vi "试剂余量显示UI.vi"() -> ()   [LabVIEW 2016, in "斯坦道CODMn新电路板.lvlib"]
uses:
  <vilib>/Utility/miscctls.llb/LVPointTypeDef.ctl
panel:
  in  "余量 14":string
  in  "余量 13":string
  in  "余量 12":string
  in  "余量 11":string
  in  "余量 10":string
  in  "余量 9":string
  in  "余量 8":string
  in  "余量 7":string
  in  "余量 6":string
  in  "余量 5":string
  in  "余量 4":string
  in  "余量 3":string
  in  "余量 2":string
  in  "余量":string
  in  "关闭":bool
  in  "全部重置":bool
  in  "试剂容量设置":bool
  in  "试剂名称设置":bool
  in  "重置 14":bool
  out "试剂 14":dbl(slide) caption="V9-2.试剂14" scale=0.0..100.0 scale format="%#_f %%"
  in  "重置 13":bool
  out "试剂 13":dbl(slide) caption="V9-1.试剂13" scale=0.0..100.0 scale format="%#_f %%"
  in  "重置 12":bool
  out "试剂 12":dbl(slide) caption="V12.试剂12" scale=0.0..100.0 scale format="%#_f %%"
  in  "重置 11":bool
  out "试剂 11":dbl(slide) caption="V11.试剂11" scale=0.0..100.0 scale format="%#_f %%"
  in  "重置 10":bool
  out "试剂 10":dbl(slide) caption="V10.试剂10" scale=0.0..100.0 scale format="%#_f %%"
  in  "重置 9":bool
  out "试剂 9":dbl(slide) caption="V9.试剂9" scale=0.0..100.0 scale format="%#_f %%"
  in  "重置 8":bool
  out "试剂 8":dbl(slide) caption="V8.试剂8" scale=0.0..100.0 scale format="%#_f %%"
  in  "重置 7":bool
  out "试剂 7":dbl(slide) caption="V7.试剂7" scale=0.0..100.0 scale format="%#_f %%"
  in  "重置 6":bool
  out "试剂 6":dbl(slide) caption="V6.试剂6" scale=0.0..100.0 scale format="%#_f %%"
  in  "重置 5":bool
  out "试剂 5":dbl(slide) caption="V5.试剂5" scale=0.0..100.0 scale format="%#_f %%"
  in  "重置 4":bool
  out "试剂 4":dbl(slide) caption="V4.试剂4" scale=0.0..100.0 scale format="%#_f %%"
  in  "重置 3":bool
  out "试剂 3":dbl(slide) caption="V3.试剂3" scale=0.0..100.0 scale format="%#_f %%"
  in  "重置 2":bool
  out "试剂 2":dbl(slide) caption="V2.试剂2" scale=0.0..100.0 scale format="%#_f %%"
  in  "重置":bool
  out "试剂":dbl(slide) caption="V1.试剂1" scale=0.0..100.0 scale format="%#_f %%"
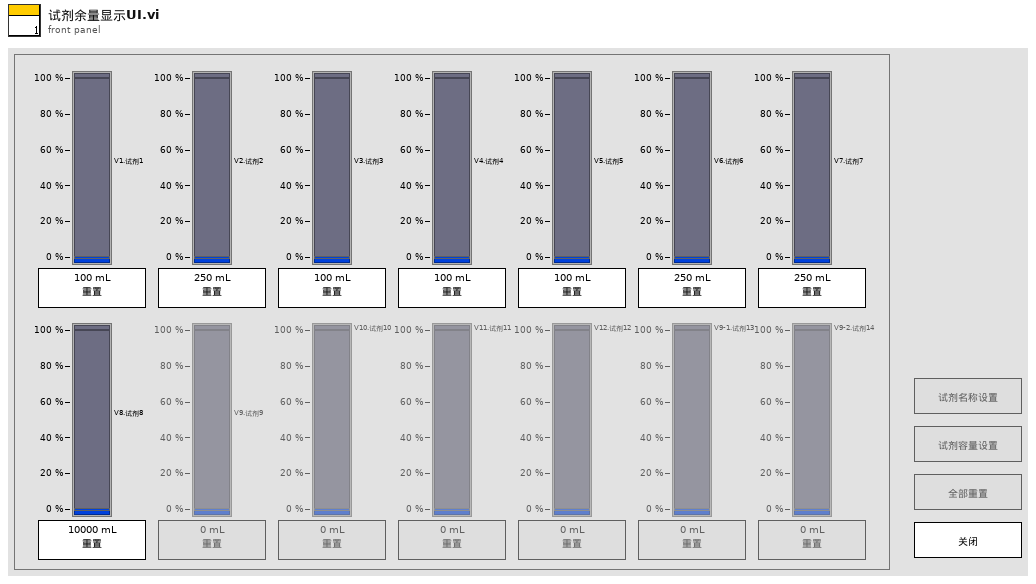
[diagram p1: front panel]
types:
  T1 = typedef "LVPointTypeDef.ctl" = cluster{"Horizontal":i16, "Vertical":i16}
  T2 = enum8{"Enabled", "Disabled", "Disabled and Grayed Out"}
  T3 = cluster{"时间标识":timestamp, "设备":string, "日志信息":string, "流程参数":string}
  T4 = cluster{"V1":sgl, "V2":sgl, "V3":sgl, "V4":sgl, "V5":sgl, "V6":sgl, "V7":sgl, "V8":sgl, "V9":sgl, "V10":sgl, "V11":sgl, "V12":sgl, "V9-1":sgl, "V9-2":sgl}
  T5 = cluster{"V":string, "V 2":string, "V 3":string, "V 4":string, "V 5":string, "V 6":string, "V 7":string, "V 8":string, "V 9":string, "V 10":string, "V 11":string, "V 12":string, "V9-1":string, "V9-2":string}
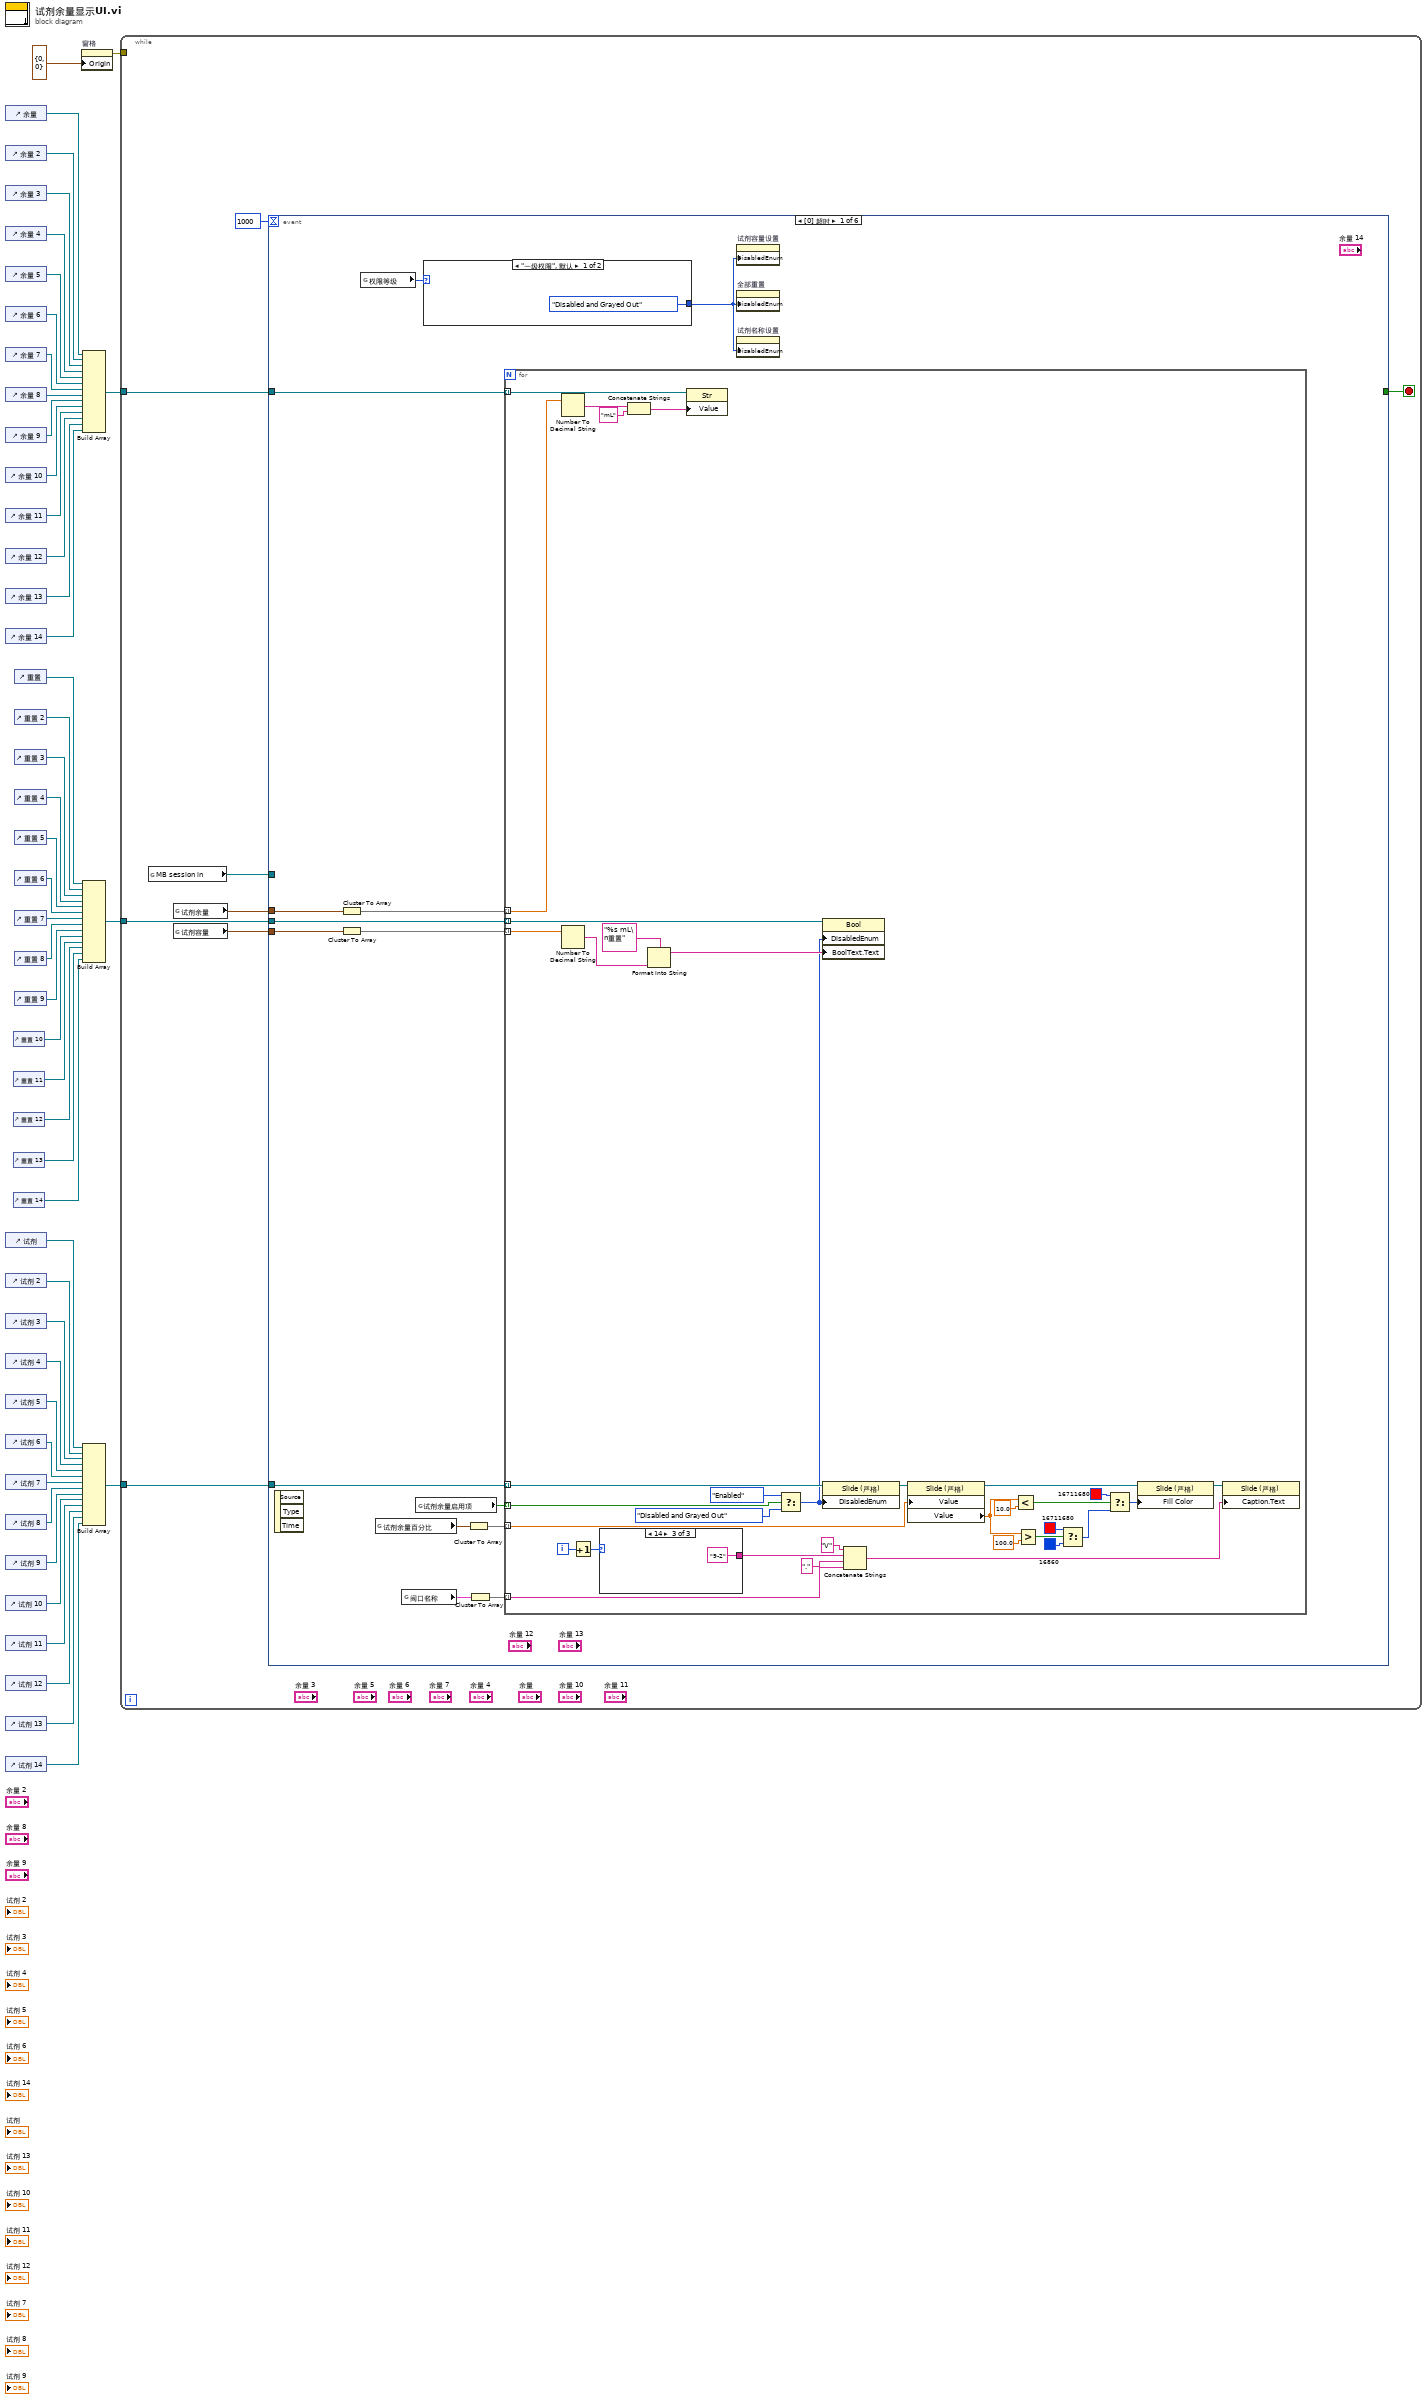
[diagram p0: block diagram]
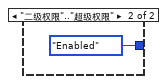
[diagram p2: hidden frame]
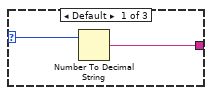
[diagram p3: hidden frame]
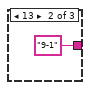
[diagram p4: hidden frame]
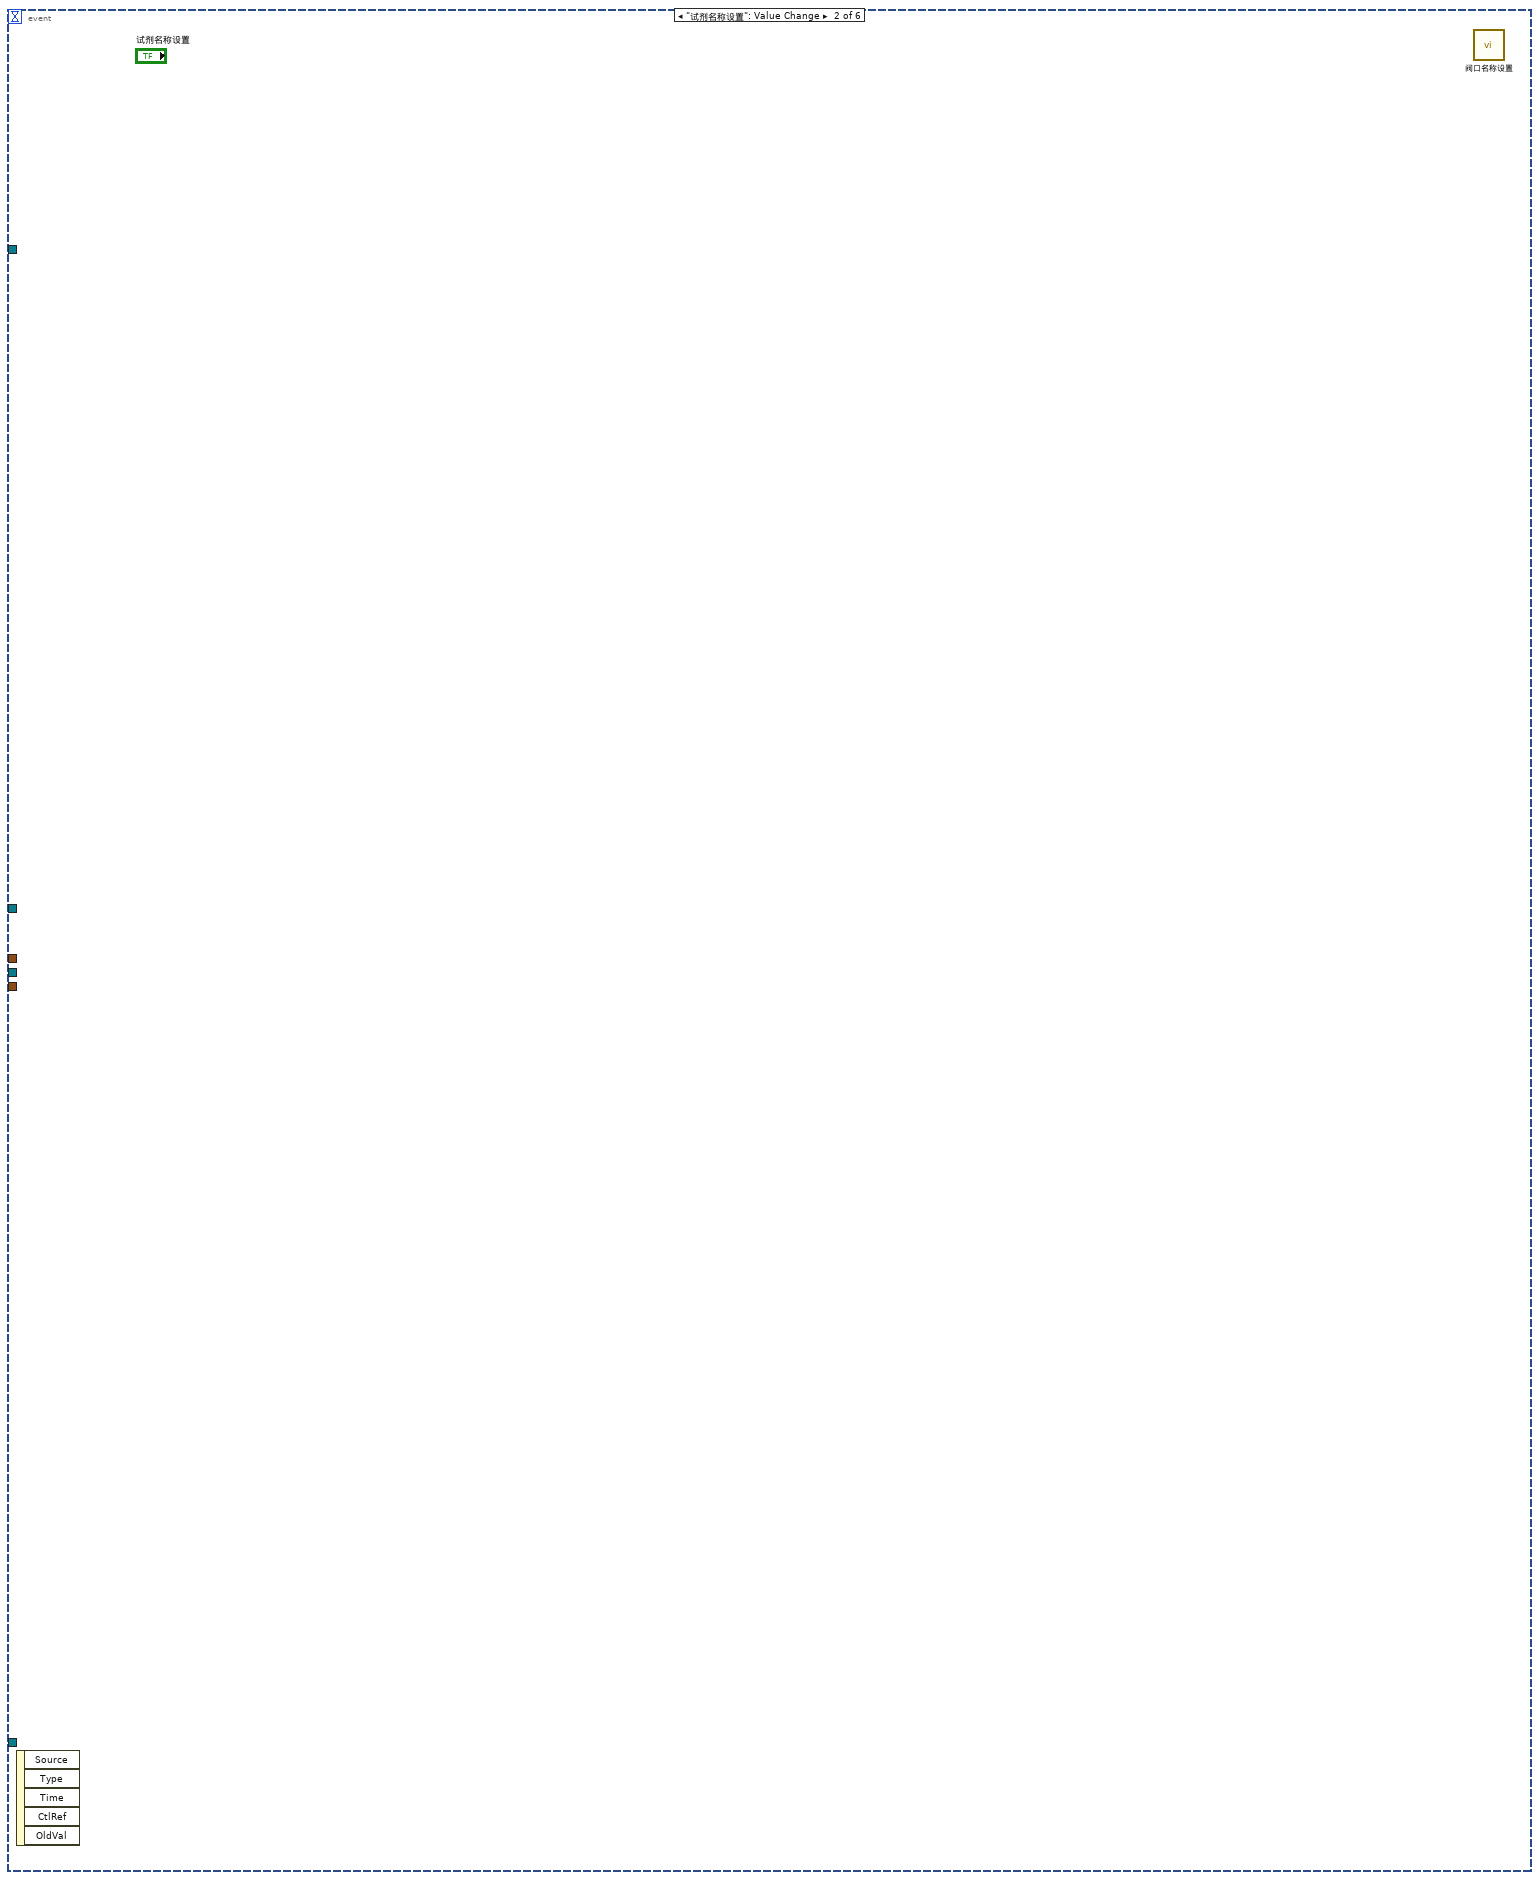
[diagram p5: hidden frame]
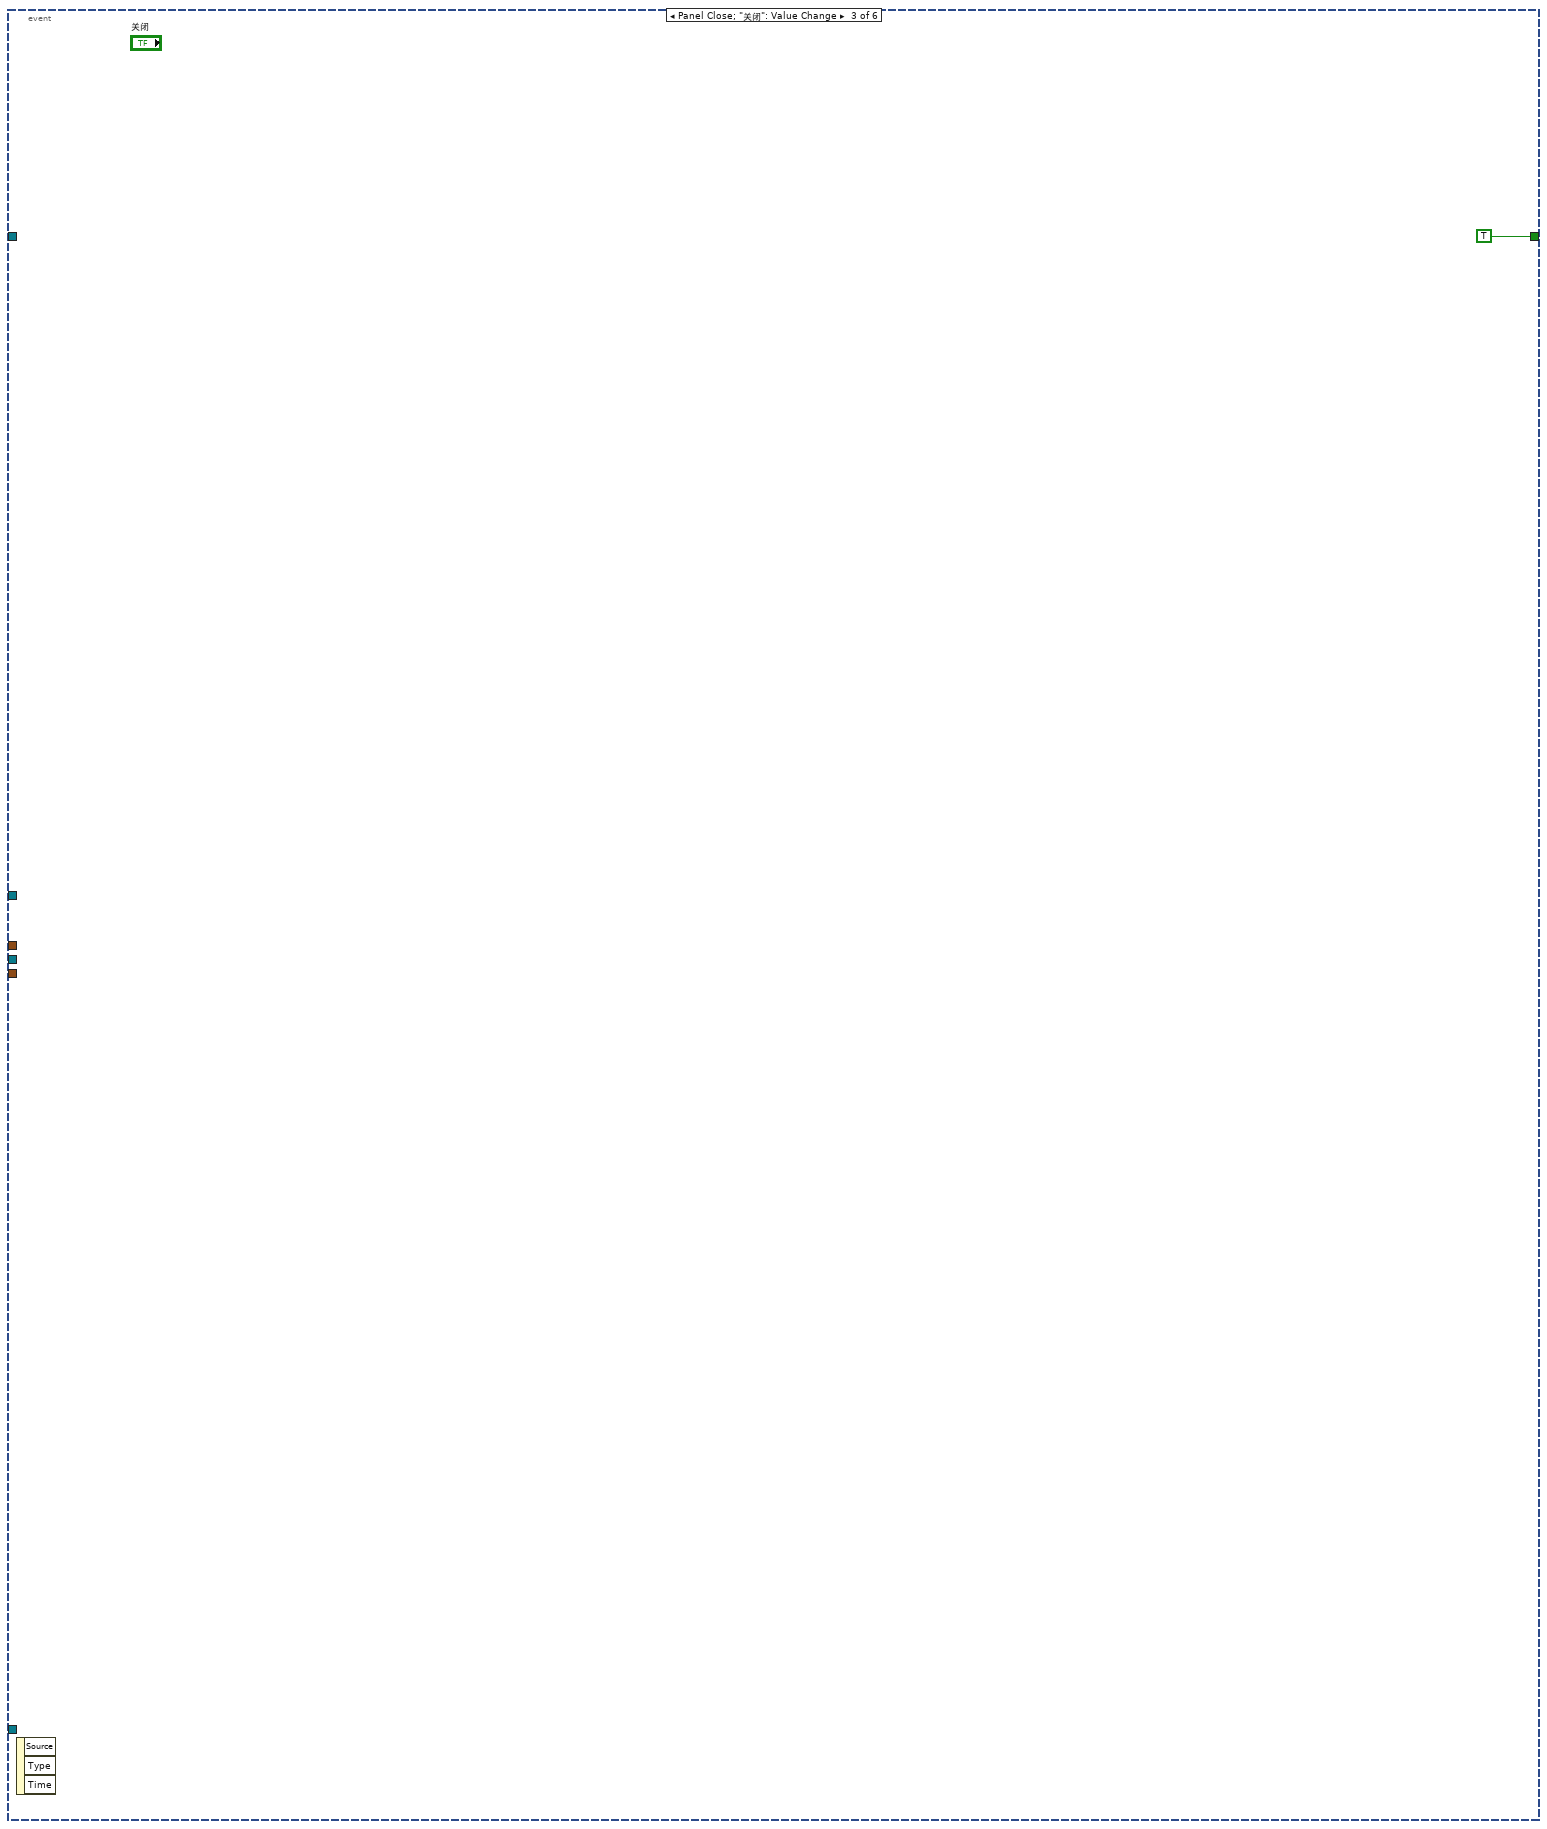
[diagram p6: hidden frame]
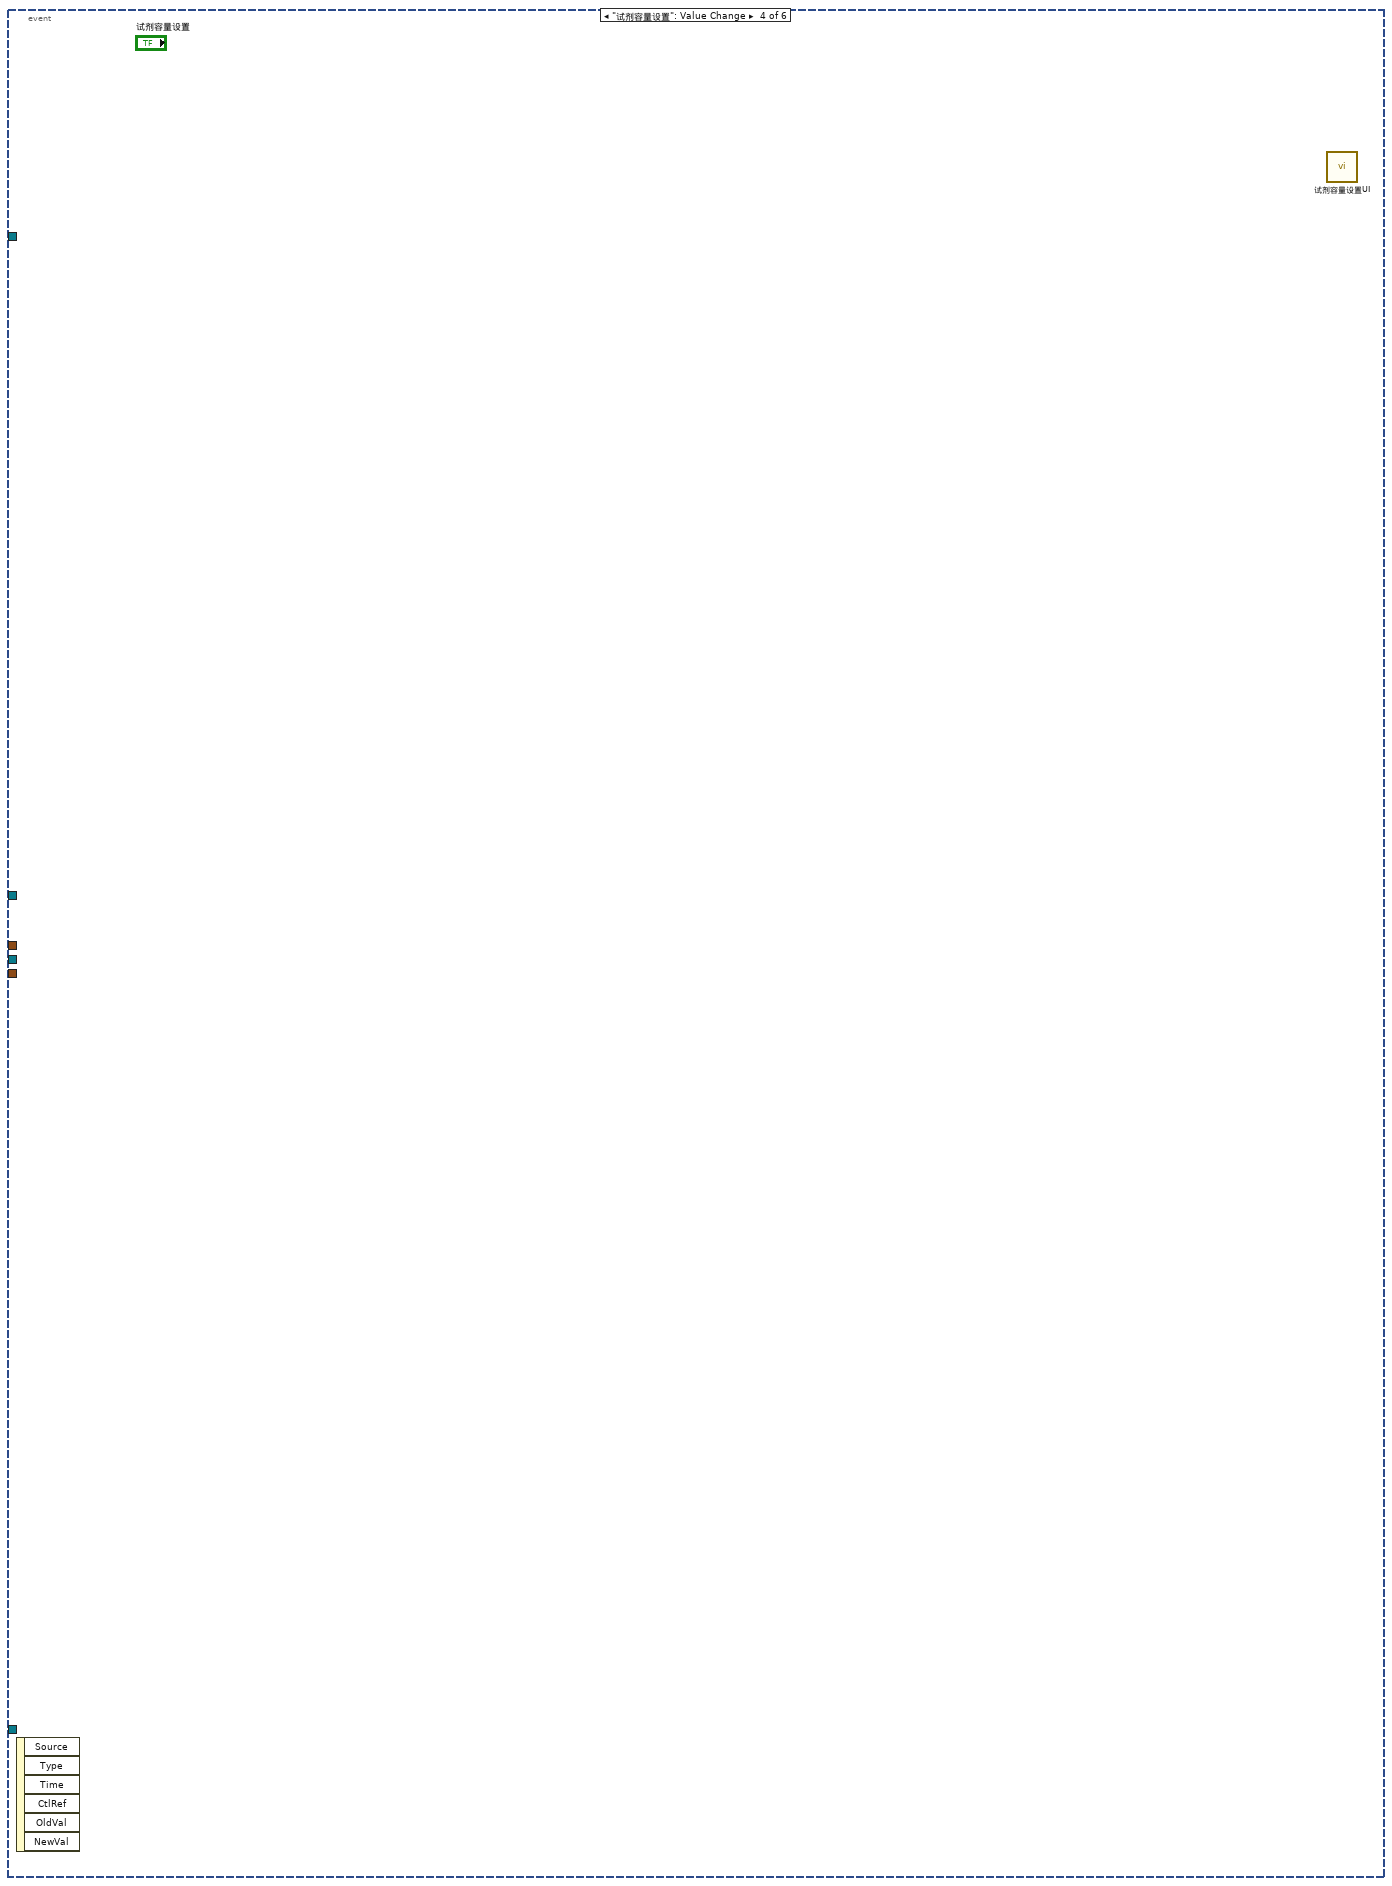
[diagram p7: hidden frame]
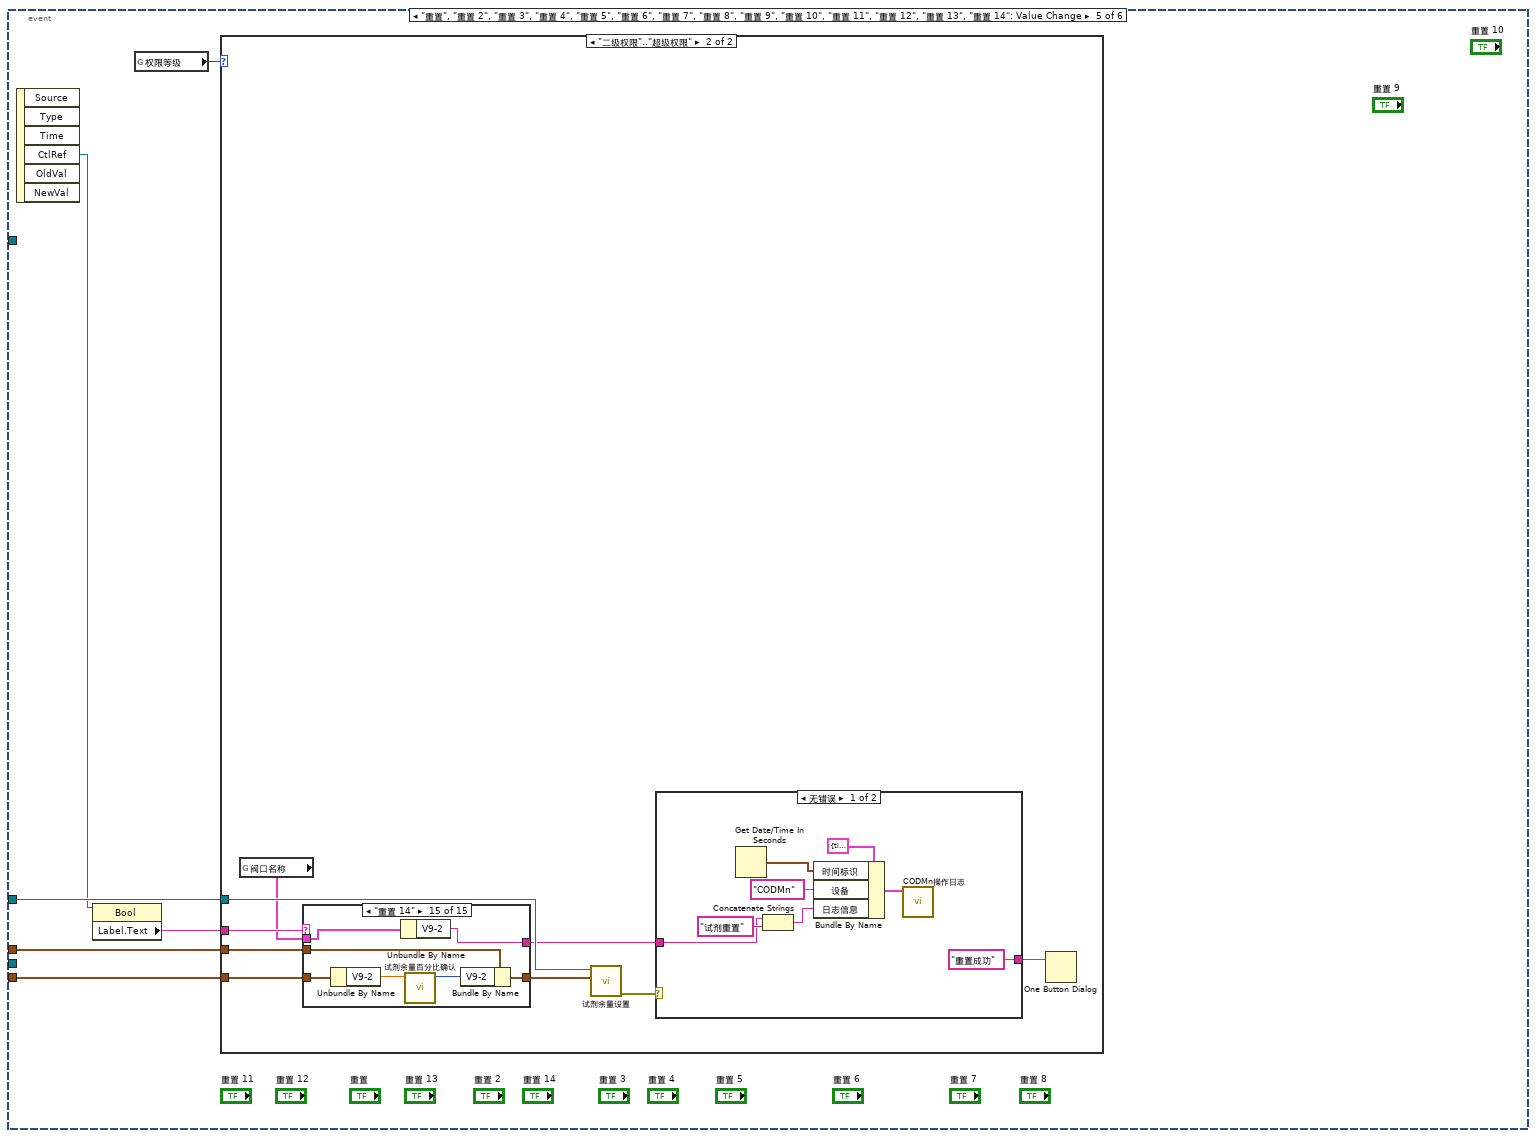
[diagram p8: hidden frame]
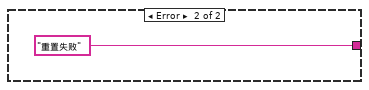
[diagram p10: hidden frame]
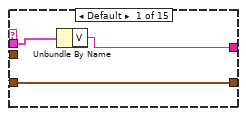
[diagram p11: hidden frame]
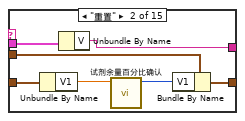
[diagram p12: hidden frame]
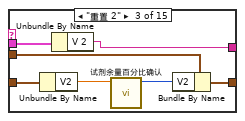
[diagram p13: hidden frame]
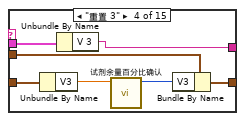
[diagram p14: hidden frame]
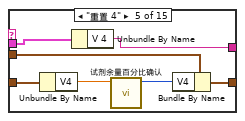
[diagram p15: hidden frame]
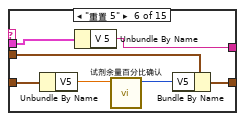
[diagram p16: hidden frame]
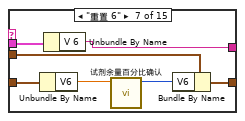
[diagram p17: hidden frame]
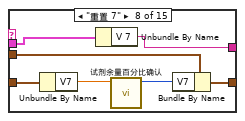
[diagram p18: hidden frame]
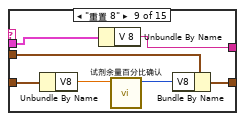
[diagram p19: hidden frame]
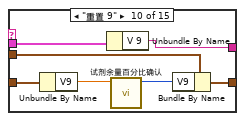
[diagram p20: hidden frame]
diagram:
  n1 = control-ref of="余量"() -> (w2:refnum<vi>)
  n2 = control-ref of="余量 2"() -> (w3:refnum<vi>)
  n3 = control-ref of="余量 3"() -> (w4:refnum<vi>)
  n4 = control-ref of="余量 4"() -> (w5:refnum<vi>)
  n5 = control-ref of="余量 5"() -> (w6:refnum<vi>)
  n6 = control-ref of="余量 6"() -> (w7:refnum<vi>)
  n7 = control-ref of="余量 7"() -> (w8:refnum<vi>)
  n8 = control-ref of="余量 8"() -> (w9:refnum<vi>)
  n9 = control-ref of="余量 9"() -> (w10:refnum<vi>)
  n10 = control-ref of="余量 10"() -> (w11:refnum<vi>)
  n11 = control-ref of="余量 11"() -> (w12:refnum<vi>)
  n12 = control-ref of="余量 12"() -> (w13:refnum<vi>)
  n13 = control-ref of="余量 13"() -> (w14:refnum<vi>)
  n14 = control-ref of="余量 14"() -> (w15:refnum<vi>)
  n15 = control-ref of="试剂"() -> (w47:refnum<vi>)
  n16 = control-ref of="试剂 2"() -> (w46:refnum<vi>)
  n17 = control-ref of="试剂 3"() -> (w45:refnum<vi>)
  n18 = control-ref of="试剂 4"() -> (w44:refnum<vi>)
  n19 = control-ref of="试剂 5"() -> (w43:refnum<vi>)
  n20 = control-ref of="试剂 6"() -> (w42:refnum<vi>)
  n21 = control-ref of="试剂 7"() -> (w41:refnum<vi>)
  n22 = control-ref of="试剂 8"() -> (w40:refnum<vi>)
  n23 = control-ref of="试剂 9"() -> (w39:refnum<vi>)
  n24 = control-ref of="试剂 10"() -> (w38:refnum<vi>)
  n25 = control-ref of="试剂 11"() -> (w37:refnum<vi>)
  n26 = control-ref of="试剂 12"() -> (w36:refnum<vi>)
  n27 = control-ref of="试剂 13"() -> (w35:refnum<vi>)
  n28 = control-ref of="试剂 14"() -> (w34:refnum<vi>)
  n29 = control-ref of="重置 10"() -> (w21:refnum<vi>)
  n30 = control-ref of="重置 11"() -> (w20:refnum<vi>)
  n31 = control-ref of="重置 12"() -> (w19:refnum<vi>)
  n32 = control-ref of="重置 13"() -> (w18:refnum<vi>)
  n33 = control-ref of="重置 14"() -> (w17:refnum<vi>)
  n34 = control-ref of="重置"() -> (w30:refnum<vi>)
  n35 = control-ref of="重置 2"() -> (w29:refnum<vi>)
  n36 = control-ref of="重置 3"() -> (w28:refnum<vi>)
  n37 = control-ref of="重置 4"() -> (w27:refnum<vi>)
  n38 = control-ref of="重置 5"() -> (w26:refnum<vi>)
  n39 = control-ref of="重置 6"() -> (w25:refnum<vi>)
  n40 = control-ref of="重置 7"() -> (w24:refnum<vi>)
  n41 = control-ref of="重置 8"() -> (w23:refnum<vi>)
  n42 = control-ref of="重置 9"() -> (w22:refnum<vi>)
  n43 = property on="窗格" class="Pane"("Origin"=T1 {"Horizontal"=0, "Vertical"=0} ("原点")) -> (error out=w31:errorcluster)  [unwired: 2 in, 1 out]
  n44 = Build Array(w2, w3, w4, w5, w6, w7, w8, w9, w10, w11, w12, w13, w14, w15) -> (w1:refnum<vi>[])
  n45 = Build Array(w30, w29, w28, w27, w26, w25, w24, w23, w22, w21, w20, w19, w18, w17) -> (w16:refnum<vi>[])
  n46 = Build Array(w47, w46, w45, w44, w43, w42, w41, w40, w39, w38, w37, w36, w35, w34) -> (w33:refnum<vi>[])
  n47 = while {
    tunnel: w33 -> [w55]
    tunnel: w31 -> [_]
    tunnel: w16 -> [w54]
    tunnel: w1 -> [w50]
    stop <- w53 stop-if-true
    n48 = global read "VARCODMn全局变量.vi" "MB session in"() -> (w51:refnum<class "MB_Master.lvclass">)
    n49 = global read "VARCODMn全局变量.vi" "试剂余量"() -> (w48:T4)
    n50 = global read "VARCODMn全局变量.vi" "试剂容量"() -> (w49:T4)
    n51 = event shown="[0] 超时" {
      selector: _ -> [_ _ _ _ _ _]
      dyn-events: _ -> [_ _ _ _ _ _]
      timeout: 1000 -> [_ _ _ _ _ _]
      tunnel: w55 -> [w69 _ _ _ _ _]
      tunnel: w54 -> [w66 _ _ _ _ _]
      tunnel: [_ _ TRUE _ _ _] -> w53
      tunnel: w49 -> [w59 _ _ _ w114 _]
      tunnel: w48 -> [w58 _ _ _ w117 _]
      tunnel: w51 -> [_ _ _ _ w118 w239]
      tunnel: w50 -> [w62 _ _ _ _ _]
      event Timeout {
        n52 = event-data() -> ()  [unwired: 1 in, 3 out]
        n53 = Cluster To Array(cluster=w58) -> (array=w63:sgl[])
        n54 = Cluster To Array(cluster=w59) -> (array=w67:sgl[])
        n55 = global read "VARCODMn全局变量.vi" "权限等级"() -> (w57:enum16{"一级权限", "二级权限", "三级权限", "超级权限"})
        n56 = global read "VARCODMn全局变量.vi" "试剂余量百分比"() -> (w60:T4)
        n57 = global read "CODMn断电保存全局变量.vi" "阀口名称"() -> (w65:T5)
        n58 = global read "VARCODMn全局变量.vi" "试剂余量启用项"() -> (w61:bool[])
        n59 = case shown="\"一级权限\", 默认" w57 {
          tunnel: [T2."Disabled and Grayed Out" ("禁用") T2."Enabled" ("禁用")] -> w56
          frame "一级权限", Default {
          }
          frame "二级权限".."超级权限" {
          }
        }
        n60 = Cluster To Array(cluster=w60) -> (array=w68:sgl[])
        n61 = Cluster To Array(cluster=w65) -> (array=w64:string[])
        n62 = for {
          tunnel: w69 -> [w101] mode=indexing
          tunnel: w68 -> [w102] mode=indexing
          tunnel: w67 -> [w90] mode=indexing
          tunnel: w66 -> [w99] mode=indexing
          tunnel: w64 -> [w96] mode=indexing
          tunnel: w63 -> [w86] mode=indexing
          tunnel: w62 -> [w85] mode=indexing
          tunnel: w61 -> [w81] mode=indexing
          i -> [w93]
          n63 = Number To Decimal String(number=w86) -> (decimal integer string=w84:string)  [unwired: 1 in]
          n64 = Number To Decimal String(number=w90) -> (decimal integer string=w89:string)  [unwired: 1 in]
          n65 = Increment(x=w93) -> (x+1=w92:i32)
          n66 = case shown="14" w92 {
            selector: w92 -> [w109 _ _]
            tunnel: [w108 "9-1" "9-2"] -> w91
            frame Default {
              n67 = Number To Decimal String(number=w109) -> (decimal integer string=w108:string)  [unwired: 1 in]
            }
            frame 13 {
            }
            frame 14 {
            }
          }
          n68 = Concatenate Strings(w84, "mL" ("字符串")) -> (w83:string)
          n69 = Format Into String(format string="%s mL\n重置" ("格式字符串"), w89) -> (resulting string=w87:string)  [unwired: 2 in, 1 out]
          n70 = property class="Str"(reference=w85, "Value"=w83) -> ()  [unwired: 1 in, 2 out]
          n71 = Select(t=T2."Enabled" ("禁用"), s=w81, f=T2."Disabled and Grayed Out" ("禁用")) -> (s? t:f=w80:T2)
          n72 = property class="Bool"(reference=w99, "DisabledEnum"=w80, "BoolText.Text"=w87) -> ()  [unwired: 1 in, 2 out]
          n73 = property class="Slide (严格)"(reference=w101, "DisabledEnum"=w80) -> (reference out=w100:refnum<vi>)  [unwired: 1 in, 1 out]
          n74 = Concatenate Strings("V" ("字符串"), w91, "." ("字符串"), w96) -> (w95:string)
          n75 = property class="Slide (严格)"(reference=w100, "Value"=w102) -> (reference out=w106:refnum<vi>, "Value"=w77:dbl)  [unwired: 1 in, 1 out]
          n76 = Less?(x=w77, y=10.0) -> (x < y?=w105:bool)
          n77 = Greater?(x=w77, y=100.0) -> (0:w75:bool)
          n78 = Select(t=u32 16711680 ("滑块颜色:背景色"), s=w75, f=u32 16860 ("滑块颜色:背景色")) -> (s? t:f=w72:u32)
          n79 = Select(t=u32 16711680 ("滑块颜色:背景色"), s=w105, f=w72) -> (s? t:f=w103:u32)
          n80 = property class="Slide (严格)"(reference=w106, "Fill Color"=w103) -> (reference out=w98:refnum<vi>)  [unwired: 1 in, 1 out]
          n81 = property class="Slide (严格)"(reference=w98, "Caption.Text"=w95) -> ()  [unwired: 1 in, 2 out]
        }
        n82 = property on="试剂容量设置" class="Bool"("DisabledEnum"=w56) -> ()  [unwired: 2 in, 2 out]
        n83 = property on="全部重置" class="Bool"("DisabledEnum"=w56) -> ()  [unwired: 2 in, 2 out]
        n84 = property on="试剂名称设置" class="Bool"("DisabledEnum"=w56) -> ()  [unwired: 2 in, 2 out]
      }
      event "试剂名称设置": Value Change {
        n85 = event-data() -> ()  [unwired: 1 in, 5 out]
        n86 = call "阀口名称设置.vi"() -> ()  [unwired: 12 in]
      }
      event Panel Close; "关闭": Value Change {
        n87 = event-data() -> ()  [unwired: 1 in, 3 out]
      }
      event "试剂容量设置": Value Change {
        n88 = event-data() -> ()  [unwired: 1 in, 6 out]
        n89 = call "试剂容量设置UI.vi"() -> ()  [unwired: 12 in]
      }
      event "重置", "重置 2", "重置 3", "重置 4", "重置 5", "重置 6", "重置 7", "重置 8", "重置 9", "重置 10", "重置 11", "重置 12", "重置 13", "重置 14": Value Change {
        n90 = event-data() -> ("CtlRef"=w116:refnum<vi>)  [unwired: 1 in, 5 out]
        n91 = property class="Bool"(reference=w116) -> ("Label.Text"=w115:string)  [unwired: 1 in, 2 out]
        n92 = global read "VARCODMn全局变量.vi" "权限等级"() -> (w113:enum16{"一级权限", "二级权限", "三级权限", "超级权限"})
        n93 = case shown="\"二级权限\"..\"超级权限\"" w113 {
          tunnel: w118 -> [_ w127]
          tunnel: w117 -> [_ w126]
          tunnel: w115 -> [_ w124]
          tunnel: w114 -> [_ w123]
          frame "一级权限", Default {
          }
          frame "二级权限".."超级权限" {
            n94 = global read "CODMn断电保存全局变量.vi" "阀口名称"() -> (w120:T5)
            n95 = case shown="\"重置 14\"" w124 {
              tunnel: w126 -> [w139 w146 w153 w160 w167 w174 w181 w188 w195 w202 w209 w216 w223 w230 w237]
              tunnel: [w139 w145 w152 w159 w166 w173 w180 w187 w194 w201 w208 w215 w222 w229 w236] -> w125
              tunnel: w123 -> [_ w144 w151 w158 w165 w172 w179 w186 w193 w200 w207 w214 w221 w228 w235]
              tunnel: w120 -> [w138 w141 w148 w155 w162 w169 w176 w183 w190 w197 w204 w211 w218 w225 w232]
              tunnel: [w137 w140 w147 w154 w161 w168 w175 w182 w189 w196 w203 w210 w217 w224 w231] -> w119
              frame Default {
                n96 = Unbundle By Name(w138) -> ("V"=w137:string)
              }
              frame "重置" {
                n97 = Unbundle By Name(w144) -> ("V1"=w143:sgl)
                n98 = Unbundle By Name(w141) -> ("V"=w140:string)
                n99 = call "试剂余量百分比确认.vi"("试剂余量百分比 2"=w143) -> ("Value"=w142:u16)  [unwired: 10 in]
                n100 = Bundle By Name(cluster=w146, "V1"=w142) -> (w145:T4)
              }
              frame "重置 2" {
                n101 = Unbundle By Name(w151) -> ("V2"=w150:sgl)
                n102 = Unbundle By Name(w148) -> ("V 2"=w147:string)
                n103 = call "试剂余量百分比确认.vi"("试剂余量百分比 2"=w150) -> ("Value"=w149:u16)  [unwired: 10 in]
                n104 = Bundle By Name(cluster=w153, "V2"=w149) -> (w152:T4)
              }
              frame "重置 3" {
                n105 = Unbundle By Name(w158) -> ("V3"=w157:sgl)
                n106 = Unbundle By Name(w155) -> ("V 3"=w154:string)
                n107 = call "试剂余量百分比确认.vi"("试剂余量百分比 2"=w157) -> ("Value"=w156:u16)  [unwired: 10 in]
                n108 = Bundle By Name(cluster=w160, "V3"=w156) -> (w159:T4)
              }
              frame "重置 4" {
                n109 = Unbundle By Name(w165) -> ("V4"=w164:sgl)
                n110 = Unbundle By Name(w162) -> ("V 4"=w161:string)
                n111 = call "试剂余量百分比确认.vi"("试剂余量百分比 2"=w164) -> ("Value"=w163:u16)  [unwired: 10 in]
                n112 = Bundle By Name(cluster=w167, "V4"=w163) -> (w166:T4)
              }
              frame "重置 5" {
                n113 = Unbundle By Name(w172) -> ("V5"=w171:sgl)
                n114 = Unbundle By Name(w169) -> ("V 5"=w168:string)
                n115 = call "试剂余量百分比确认.vi"("试剂余量百分比 2"=w171) -> ("Value"=w170:u16)  [unwired: 10 in]
                n116 = Bundle By Name(cluster=w174, "V5"=w170) -> (w173:T4)
              }
              frame "重置 6" {
                n117 = Unbundle By Name(w179) -> ("V6"=w178:sgl)
                n118 = Unbundle By Name(w176) -> ("V 6"=w175:string)
                n119 = call "试剂余量百分比确认.vi"("试剂余量百分比 2"=w178) -> ("Value"=w177:u16)  [unwired: 10 in]
                n120 = Bundle By Name(cluster=w181, "V6"=w177) -> (w180:T4)
              }
              frame "重置 7" {
                n121 = Unbundle By Name(w186) -> ("V7"=w185:sgl)
                n122 = Unbundle By Name(w183) -> ("V 7"=w182:string)
                n123 = call "试剂余量百分比确认.vi"("试剂余量百分比 2"=w185) -> ("Value"=w184:u16)  [unwired: 10 in]
                n124 = Bundle By Name(cluster=w188, "V7"=w184) -> (w187:T4)
              }
              frame "重置 8" {
                n125 = Unbundle By Name(w193) -> ("V8"=w192:sgl)
                n126 = Unbundle By Name(w190) -> ("V 8"=w189:string)
                n127 = call "试剂余量百分比确认.vi"("试剂余量百分比 2"=w192) -> ("Value"=w191:u16)  [unwired: 10 in]
                n128 = Bundle By Name(cluster=w195, "V8"=w191) -> (w194:T4)
              }
              frame "重置 9" {
                n129 = Unbundle By Name(w200) -> ("V9"=w199:sgl)
                n130 = Unbundle By Name(w197) -> ("V 9"=w196:string)
                n131 = call "试剂余量百分比确认.vi"("试剂余量百分比 2"=w199) -> ("Value"=w198:u16)  [unwired: 10 in]
                n132 = Bundle By Name(cluster=w202, "V9"=w198) -> (w201:T4)
              }
              frame "重置 10" {
                n133 = Unbundle By Name(w207) -> ("V10"=w206:sgl)
                n134 = Unbundle By Name(w204) -> ("V 10"=w203:string)
                n135 = call "试剂余量百分比确认.vi"("试剂余量百分比 2"=w206) -> ("Value"=w205:u16)  [unwired: 10 in]
                n136 = Bundle By Name(cluster=w209, "V10"=w205) -> (w208:T4)
              }
              frame "重置 11" {
                n137 = Unbundle By Name(w214) -> ("V11"=w213:sgl)
                n138 = call "试剂余量百分比确认.vi"("试剂余量百分比 2"=w213) -> ("Value"=w212:u16)  [unwired: 10 in]
                n139 = Unbundle By Name(w211) -> ("V 11"=w210:string)
                n140 = Bundle By Name(cluster=w216, "V11"=w212) -> (w215:T4)
              }
              frame "重置 12" {
                n141 = Unbundle By Name(w221) -> ("V12"=w220:sgl)
                n142 = call "试剂余量百分比确认.vi"("试剂余量百分比 2"=w220) -> ("Value"=w219:u16)  [unwired: 10 in]
                n143 = Unbundle By Name(w218) -> ("V 12"=w217:string)
                n144 = Bundle By Name(cluster=w223, "V12"=w219) -> (w222:T4)
              }
              frame "重置 13" {
                n145 = Unbundle By Name(w228) -> ("V9-1"=w227:sgl)
                n146 = call "试剂余量百分比确认.vi"("试剂余量百分比 2"=w227) -> ("Value"=w226:u16)  [unwired: 10 in]
                n147 = Unbundle By Name(w225) -> ("V9-1"=w224:string)
                n148 = Bundle By Name(cluster=w230, "V9-1"=w226) -> (w229:T4)
              }
              frame "重置 14" {
                n149 = Unbundle By Name(w235) -> ("V9-2"=w234:sgl)
                n150 = Unbundle By Name(w232) -> ("V9-2"=w231:string)
                n151 = call "试剂余量百分比确认.vi"("试剂余量百分比 2"=w234) -> ("Value"=w233:u16)  [unwired: 10 in]
                n152 = Bundle By Name(cluster=w237, "V9-2"=w233) -> (w236:T4)
              }
            }
            n153 = call "试剂余量设置.vi"("试剂余量"=w125, "MB session in"=w127) -> ("error out"=w122:errorcluster)  [unwired: 8 in, 1 out]
            n154 = case shown="无错误" w122 {
              tunnel: ["重置成功" ("消息") "重置失败" ("消息")] -> w121
              tunnel: w119 -> [w128 _]
              frame No Error {
                n155 = Get Date/Time In Seconds() -> (seconds since 1Jan1904=w131:timestamp)
                n156 = Concatenate Strings(w128, "试剂重置" ("字符串")) -> (w134:string)
                n157 = Bundle By Name(cluster=T3 {"时间标识"=timestamp(0 s since 1904-01-01), "设备"="", "日志信息"="", "流程参数"=""} ("data in"), "时间标识"=w131, "设备"="CODMn", "日志信息"=w134) -> (w130:T3)
                n158 = call "CODMn操作日志.vi"("data in"=w130) -> ()  [unwired: 11 in]
              }
              frame Error {
              }
            }
            n159 = One Button Dialog(message=w121) -> ()  [unwired: 1 in, 1 out]
          }
        }
      }
      event "全部重置": Value Change {
        n160 = event-data() -> ()  [unwired: 1 in, 6 out]
        n161 = global read "VARCODMn全局变量.vi" "权限等级"() -> (w238:enum16{"一级权限", "二级权限", "三级权限", "超级权限"})
        n162 = case shown="\"二级权限\"..\"超级权限\"" w238 {
          tunnel: w239 -> [_ w242]
          frame "一级权限", Default {
          }
          frame "二级权限".."超级权限" {
            n163 = call "试剂余量重置.vi"("MB session in"=w242) -> ("error out"=w240:errorcluster)  [unwired: 9 in, 1 out]
            n164 = case shown="无错误" w240 {
              tunnel: ["重置成功" ("消息") "重置失败" ("消息")] -> w241
              frame No Error {
                n165 = Get Date/Time In Seconds() -> (seconds since 1Jan1904=w246:timestamp)
                n166 = Concatenate Strings("所有" ("字符串"), "试剂重置" ("字符串")) -> (w249:string)
                n167 = Bundle By Name(cluster=T3 {"时间标识"=timestamp(0 s since 1904-01-01), "设备"="", "日志信息"="", "流程参数"=""} ("data in"), "时间标识"=w246, "设备"="CODMn", "日志信息"=w249) -> (w245:T3)
                n168 = call "CODMn操作日志.vi"("data in"=w245) -> ()  [unwired: 11 in]
              }
              frame Error {
              }
            }
            n169 = One Button Dialog(message=w241) -> ()  [unwired: 1 in, 1 out]
          }
        }
      }
    }
  }
